vi "Sequence.BuildPreviewWaveform.vi"(7 "WaveformGraph in":refnum<vi>, 8 "error in (no error)":errorcluster, 10 "Rows":cluster{"Start Index":i32, "Length":i32}={"Start Index"=0, "Length"=-1}, 11 "input cluster":T1) -> (0 "error out":errorcluster, 2 "Wavefrom":waveform(dbl)[](array[waveform]), 3 "input cluster out":T1)   [LabVIEW 2013, in "Simple Sequence Editor.lvlib"]
uses:
  Simple Sequence Editor.lvlib
  Types/StateVariables.ctl
  Types/ChannelProperties.ctl
  <vilib>/Analysis/1siggen.llb/Ramp Pattern by Samples.vi
  <vilib>/Analysis/1siggen.llb/Ramp Pattern by Delta.vi
  <vilib>/Analysis/NI_AALBase.lvlib
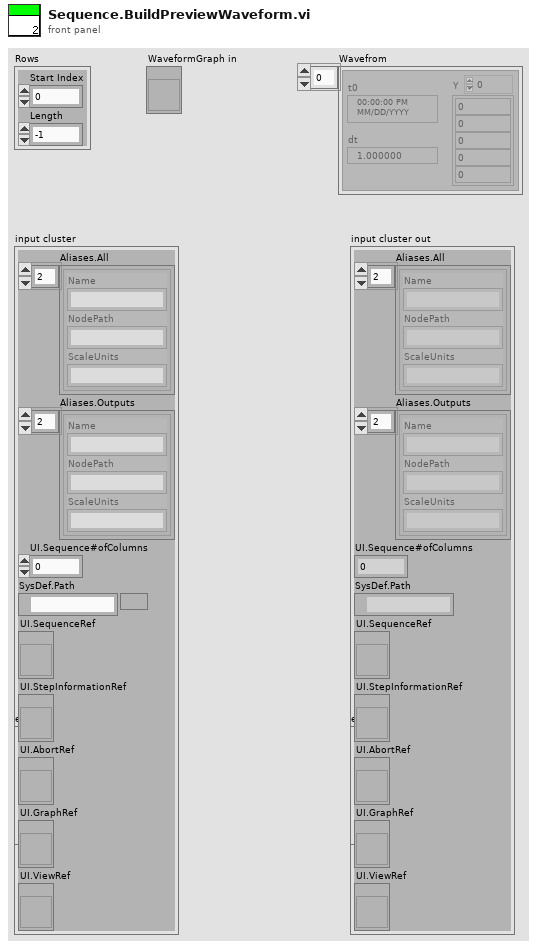
[diagram p1: front panel]
types:
  T1 = typedef "Simple Sequence Editor.lvlib/StateVariables.ctl" = cluster{"Aliases.All":T2[], "Aliases.Outputs":T2[], "UI.Sequence#ofColumns":i32, "SysDef.Path":path, "UI.SequenceRef":refnum<vi>, "UI.StepInformationRef":refnum<vi>, "UI.AbortRef":refnum<vi>, "UI.GraphRef":refnum<vi>, "UI.ViewRef":refnum<vi>}
  T2 = typedef "Simple Sequence Editor.lvlib/ChannelProperties.ctl" = cluster{"Name":string, "NodePath":string, "ScaleUnits":string}
  T3 = typedef "Simple Sequence Editor.lvlib/StepTypes.ctl" = enum8{"Step", "iStep", "Ramp", "Unchanged", "Unknown"}
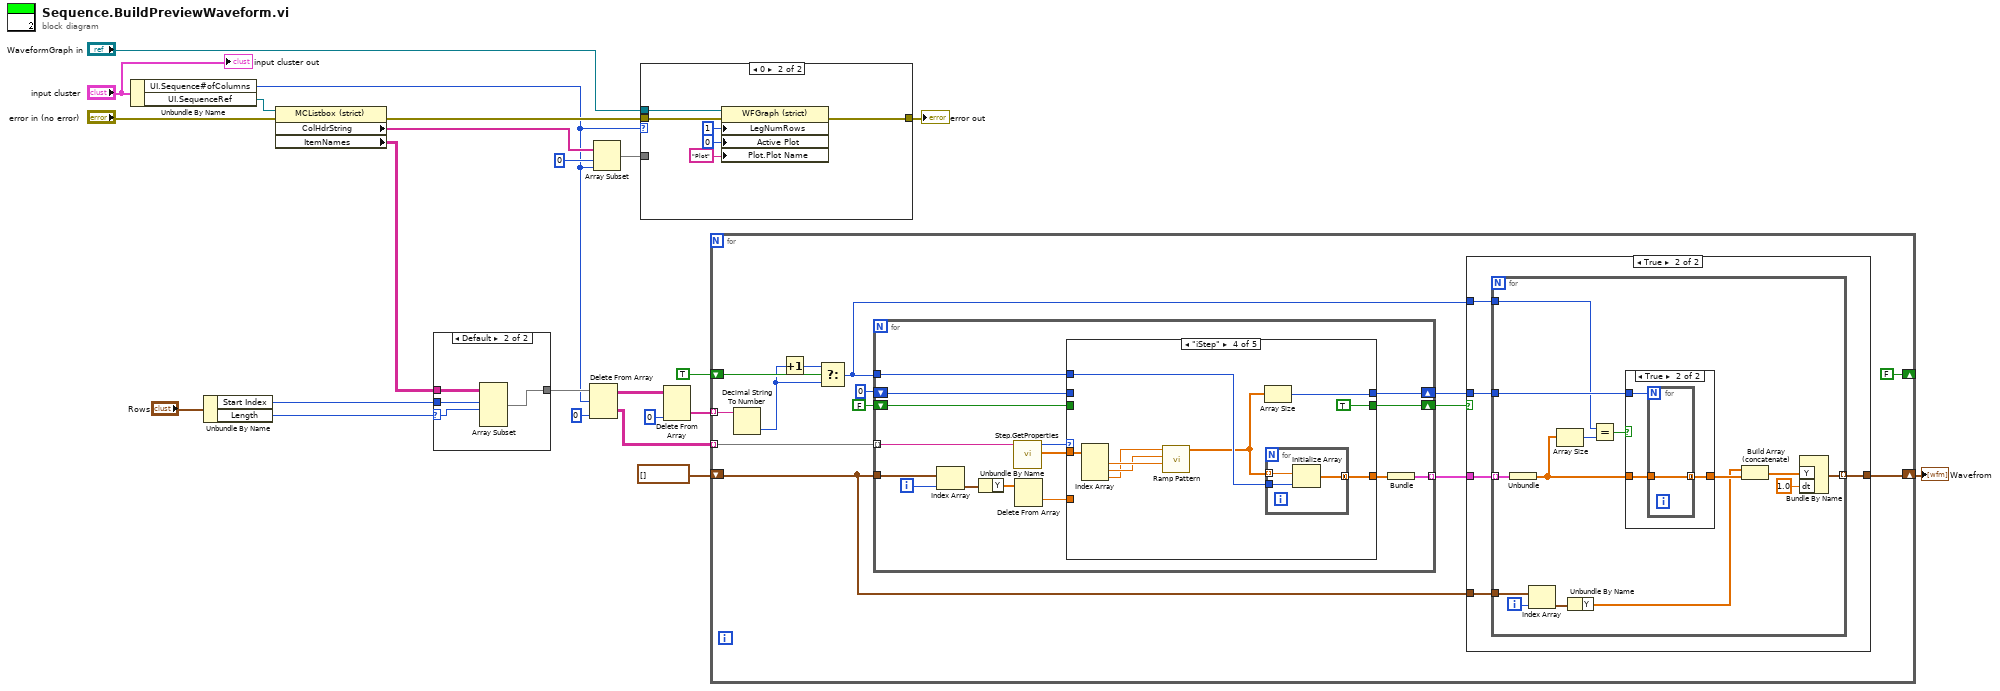
[diagram p0: block diagram]
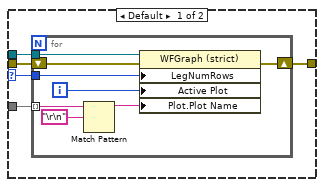
[diagram p2: hidden frame]
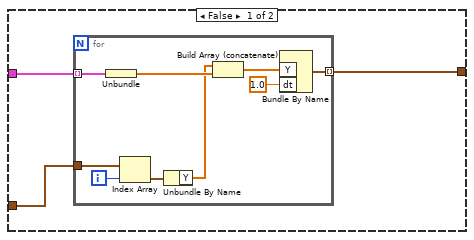
[diagram p4: hidden frame]
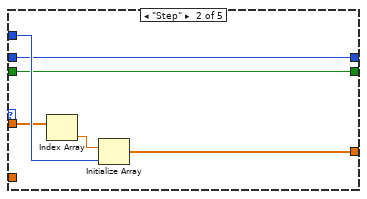
[diagram p7: hidden frame]
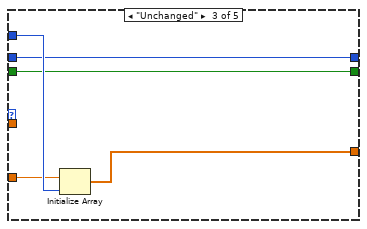
[diagram p8: hidden frame]
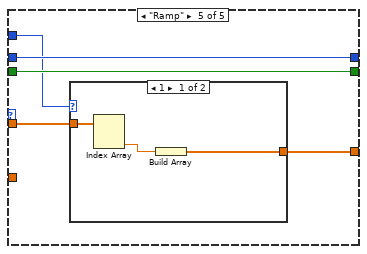
[diagram p9: hidden frame]
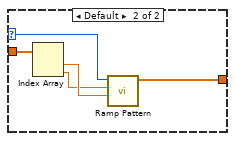
[diagram p10: hidden frame]
diagram:
  n1 = Unbundle By Name("input cluster") -> ("UI.Sequence#ofColumns"=w1:i32, "UI.SequenceRef"=w13:refnum<vi>)
  n2 = Unbundle By Name("Rows") -> ("Start Index"=w4:i32, "Length"=w7:i32)
  n3 = property class="MCListbox (strict)"(reference=w13, error in="error in (no error)") -> (error out=w9:errorcluster, "ColHdrString"=w11:string[], "ItemNames"=w6:string[][])  [unwired: 1 out]
  n4 = case shown="Default" w7 {
    selector: w7 -> [_ w25]
    tunnel: w6 -> [w24 w28]
    tunnel: [w24 w27] -> w5
    tunnel: w4 -> [_ w26]
    frame -1 {
    }
    frame Default {
      n5 = Array Subset(array=w28, index (row)=w26, length (row)=w25) -> (w27:string[][])  [unwired: 2 in]
    }
  }
  n6 = Delete From Array(array=w5, length=w1, index (col)=0 ("disabled index (col)")) -> (deleted portion=w3:string[][], array with subset deleted=w17:string[][])  [unwired: 1 in]
  n7 = Array Subset(array=w11, index=0, length=w1) -> (w22:string[])
  n8 = case shown="0" w1 {
    selector: w1 -> [w29 _]
    tunnel: [w33 w47] -> w23
    tunnel: w22 -> [w32 _]
    tunnel: "WaveformGraph in" -> [w31 w46]
    tunnel: w9 -> [w30 w45]
    frame Default {
      n9 = for {
        tunnel: w29 -> [w41]
        tunnel: w32 -> [w38] mode=indexing
        shift-right: [w35] -> w33
        shift-left: w30 -> [w36]
        tunnel: w31 -> [w34]
        i -> [w40]
        n10 = Match Pattern(string=w38, regular expression="\r\n") -> (before substring=w39:string)  [unwired: 1 in, 3 out]
        n11 = property on="Property Node" class="WFGraph (strict)"(reference=w34, error in=w36, "LegNumRows"=w41, "Active Plot"=w40, "Plot.Plot Name"=w39) -> (error out=w35:errorcluster)  [unwired: 1 out]
      }
    }
    frame 0 {
      n12 = property on="Property Node" class="WFGraph (strict)"(reference=w46, error in=w45, "LegNumRows"=u32 1 ("Legend:Number of Rows"), "Active Plot"=u32 0, "Plot.Plot Name"="Plot") -> (error out=w47:errorcluster)  [unwired: 1 out]
    }
  }
  "error out" <- w23
  n13 = Delete From Array(array=w17, index (col)=0 ("disabled index (col)")) -> (deleted portion=w2:string[])  [unwired: 2 in, 1 out]
  n14 = for {
    tunnel: w3 -> [w61] mode=indexing
    tunnel: w2 -> [w60] mode=indexing
    shift-right: [FALSE] -> _
    shift-left: TRUE -> [w53]
    shift-right: [w49] -> w20
    shift-left: waveform(dbl)[] [] -> [w48]
    n15 = Decimal String To Number(string=w60) -> (number=w52:i32)  [unwired: 2 in, 1 out]
    n16 = Increment(x=w52) -> (x+1=w51:i32)
    n17 = Select(t=w51, s=w53, f=w52) -> (s? t:f=w50:i32)
    n18 = for {
      tunnel: w61 -> [w112] mode=indexing
      tunnel: w50 -> [w110]
      shift-right: [w107] -> w57
      shift-left: FALSE -> [w108]
      shift-right: [w105] -> w56
      shift-left: 0 -> [w104]
      tunnel: [w103] -> w55 mode=indexing
      tunnel: w48 -> [w102]
      i -> [w100]
      n19 = Index Array(array=w102, index=w100) -> (element=w99:waveform(dbl))
      n20 = Unbundle By Name(w99) -> ("Y"=w98:dbl[])
      n21 = call "Step.GetProperties.vi"("String in"=w112) -> ("Parameters"=w109:dbl[], "Step"=w111:T3)  [unwired: 9 in]
      n22 = Delete From Array(array=w98) -> (deleted portion=w101:dbl)  [unwired: 2 in, 1 out]
      n23 = case shown="\"iStep\"" w111 {
        tunnel: w110 -> [_ w120 w125 w133 w138]
        tunnel: w109 -> [_ w119 _ w134 w142]
        tunnel: [_ w117 w124 w128 w141] -> w106
        tunnel: w108 -> [w114 w116 w123 _ w140]
        tunnel: [w114 w116 w123 TRUE w140] -> w107
        tunnel: [w113 w115 w122 w126 w139] -> w105
        tunnel: w104 -> [w113 w115 w122 _ w139]
        tunnel: w101 -> [_ _ w121 _ _]
        frame Default {
        }
        frame "Step" {
          n24 = Index Array(array=w119) -> (element=w118:dbl)  [unwired: 1 in]
          n25 = Initialize Array(w118, w120) -> (w117:dbl[])
        }
        frame "Unchanged" {
          n26 = Initialize Array(w121, w125) -> (w124:dbl[])
        }
        frame "iStep" {
          n27 = Index Array(array=w134) -> (element #1=w132:dbl, element #2=w131:dbl, element #3=w130:dbl)  [unwired: 3 in]
          n28 = call-poly <vilib>:"Ramp Pattern.vi"("start"=w132, "end"=w131, "delta"=w130) -> ("Ramp Pattern"=w127:dbl[])  [unwired: 6 in, 2 out]
          n29 = Array Size(array=w127) -> (size(s)=w126:i32)
          n30 = for {
            tunnel: w133 -> [w137]
            tunnel: w127 -> [w136] mode=indexing
            tunnel: [w135] -> w128 mode=concatenating
            n31 = Initialize Array(w136, w137) -> (w135:dbl[])
          }
        }
        frame "Ramp" {
          n32 = case shown="1" w138 {
            selector: w138 -> [_ w146]
            tunnel: w142 -> [w145 w150]
            tunnel: [w143 w147] -> w141
            frame 1 {
              n33 = Index Array(array=w145) -> (element #2=w144:dbl)  [unwired: 2 in, 1 out]
              n34 = Build Array(w144) -> (w143:dbl[])
            }
            frame Default {
              n35 = Index Array(array=w150) -> (element #1=w149:dbl, element #2=w148:dbl)  [unwired: 2 in]
              n36 = call-poly <vilib>:"Ramp Pattern.vi"("start"=w149, "end"=w148, "samples"=w146) -> ("Ramp Pattern"=w147:dbl[])  [unwired: 7 in, 1 out]
            }
          }
        }
      }
      n37 = Bundle("Ramp Pattern"=w106) -> (w103:cluster{"Ramp Pattern":dbl[]})  [unwired: 1 in]
    }
    n38 = case shown="True" w57 {
      tunnel: w56 -> [_ w77]
      tunnel: w55 -> [w64 w78]
      tunnel: w50 -> [_ w76]
      tunnel: [w63 w75] -> w49
      tunnel: w48 -> [w62 w74]
      frame False {
        n39 = for {
          tunnel: w64 -> [w73] mode=indexing
          tunnel: [w71] -> w63 mode=indexing
          tunnel: w62 -> [w66]
          i -> [w67]
          n40 = Unbundle(w73) -> ("Ramp Pattern"=w70:dbl[])
          n41 = Index Array(array=w66, index=w67) -> (element=w65:waveform(dbl))
          n42 = Unbundle By Name(w65) -> ("Y"=w68:dbl[])
          n43 = Build Array (concatenate)(w68, w70) -> (w69:dbl[])
          n44 = Bundle By Name("Y"=w69, "dt"=1.0) -> (w71:waveform(dbl))  [unwired: 1 in]
        }
      }
      frame True {
        n45 = for {
          tunnel: w78 -> [w91] mode=indexing
          tunnel: w77 -> [w92]
          tunnel: w76 -> [w88]
          tunnel: [w85] -> w75 mode=indexing
          tunnel: w74 -> [w80]
          i -> [w81]
          n46 = Unbundle(w91) -> ("Ramp Pattern"=w90:dbl[])
          n47 = Index Array(array=w80, index=w81) -> (element=w79:waveform(dbl))
          n48 = Array Size(array=w90) -> (size(s)=w89:i32)
          n49 = Unbundle By Name(w79) -> ("Y"=w82:dbl[])
          n50 = Equal?(x=w88, y=w89) -> (x = y?=w87:bool)
          n51 = case shown="True" w87 {
            tunnel: w92 -> [_ w96]
            tunnel: w90 -> [w93 w95]
            tunnel: [w93 w94] -> w84
            frame False {
            }
            frame True {
              n52 = for {
                N: w96 -> [_]
                tunnel: w95 -> [w97]
                tunnel: [w97] -> w94 mode=concatenating
              }
            }
          }
          n53 = Build Array (concatenate)(w82, w84) -> (w83:dbl[])
          n54 = Bundle By Name("Y"=w83, "dt"=1.0) -> (w85:waveform(dbl))  [unwired: 1 in]
        }
      }
    }
  }
  "Wavefrom" <- w20
  "input cluster out" <- "input cluster"
